vi "NewFile.vi"(8 "error in (no error)":errorcluster, 10 "FileExtension":string, 11 "LogFolder":path) -> (0 "error out":errorcluster, 3 "LogfileRef Out":refnum<file>)   [LabVIEW 2016, in "Log4Lv.lvlib"]
doc: "Use this template to build a VI to use as a subVI."
uses:
  Log4Lv.lvlib
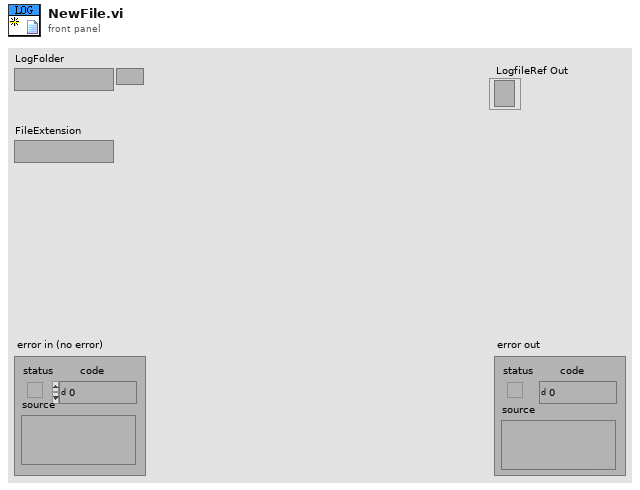
[diagram p1: front panel]
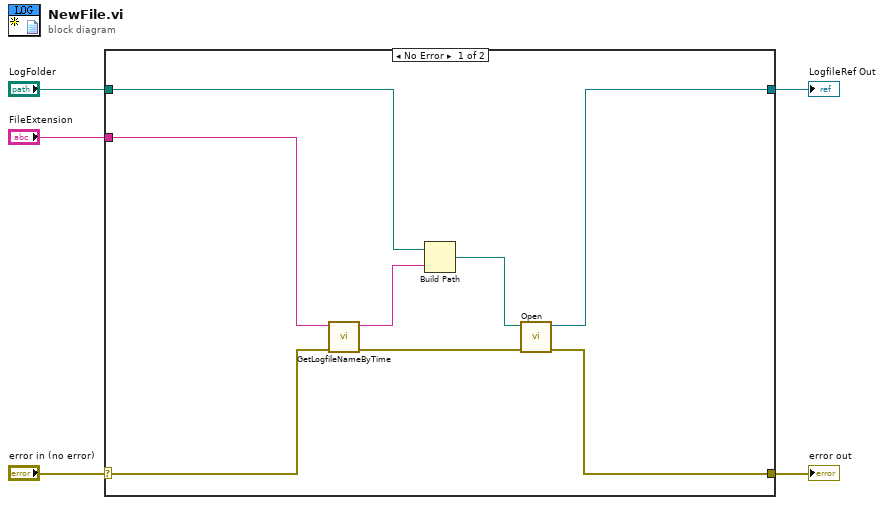
[diagram p0: block diagram]
diagram:
  n1 = case shown="No Error" "error in (no error)" {
    selector: "error in (no error)" -> [w12 w14]
    tunnel: [w11 w14] -> w4
    tunnel: "LogFolder" -> [w9 _]
    tunnel: [w7 _] -> w2
    tunnel: "FileExtension" -> [w6 _]
    frame No Error {
      n2 = call "GetLogfileNameByTime.vi"("error in (no error)"=w12, "FileExtension"=w6) -> ("error out"=w10:errorcluster, "Name by Time"=w8:string)  [unwired: 8 in]
      n3 = Build Path(base path=w9, name or relative path=w8) -> (appended path=w13:path)
      n4 = call "Open.vi"("error in (no error)"=w10, "Logfile"=w13) -> ("error out"=w11:errorcluster, "Logfile Ref Out"=w7:refnum<file>)  [unwired: 8 in]
    }
    frame Error {
    }
  }
  "error out" <- w4
  "LogfileRef Out" <- w2
